vi "Get Target IP.vi"(8 "error in (no error)":errorcluster, 11 "TargetItem in":refnum<vi>) -> (0 "error out":errorcluster, 3 "string":string)   [LabVIEW 2014, in "Scan Engine editor node.lvclass"]
uses:
  Scan Engine editor node.lvclass
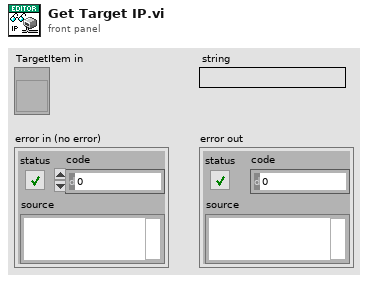
[diagram p1: front panel]
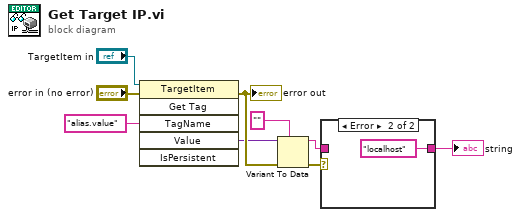
[diagram p0: block diagram]
diagram:
  n1 = invoke class="TargetItem" method="Get Tag"(reference="TargetItem in", error in="error in (no error)", "TagName"="alias.value" ("Tag Name")) -> (error out=w9:errorcluster, "Value"=w4:variant)  [unwired: 3 in, 4 out]
  "error out" <- w9
  n2 = Variant To Data(error in=w9, type="" ("Tag Name"), Variant=w4) -> (data=w6:string, error out=w8:errorcluster)
  n3 = case shown="Error" w8 {
    tunnel: [w10 "localhost" ("string")] -> w5
    tunnel: w6 -> [w10 _]
    frame No Error {
    }
    frame Error {
    }
  }
  "string" <- w5
